vi "Main.vi"() -> ()   [LabVIEW 2023]
panel:
  in  "Start":bool
  in  "Vipassana Time (min)":dbl
  in  "Anapana Time (min)":dbl
  in  "Vipassana":bool
  in  "Anapana":bool
  # "Time(minutes)"
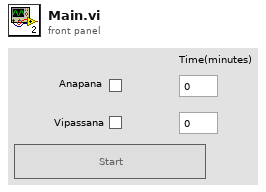
[diagram p1: front panel]
types:
  T1 = enum8{"Enabled", "Disabled", "Disabled and Grayed Out"}
  T2 = enum32{"Invalid", "Standard", "Closed", "Hidden", "Minimized", "Maximized"}
  T3 = enum32{"invalid app kind", "Development System", "Run Time System", "Student Edition", "Embedded LabVIEW", "Evaluation", "Custom"}
  T4 = cluster{"Core":cluster{"Current VI Reference":refnum<vi>, "Close Panel on Exit?":bool}, "Anapana Start Time":timestamp, "Vipassana Start Time":timestamp, "Anapana":bool, " Vipassana":bool, "Anapana Time (min)":dbl, "Vipassana Time (min)":dbl, "Real Sound?":bool}
  T5 = cluster{"Current VI Reference":refnum<vi>, "Close Panel on Exit?":bool}
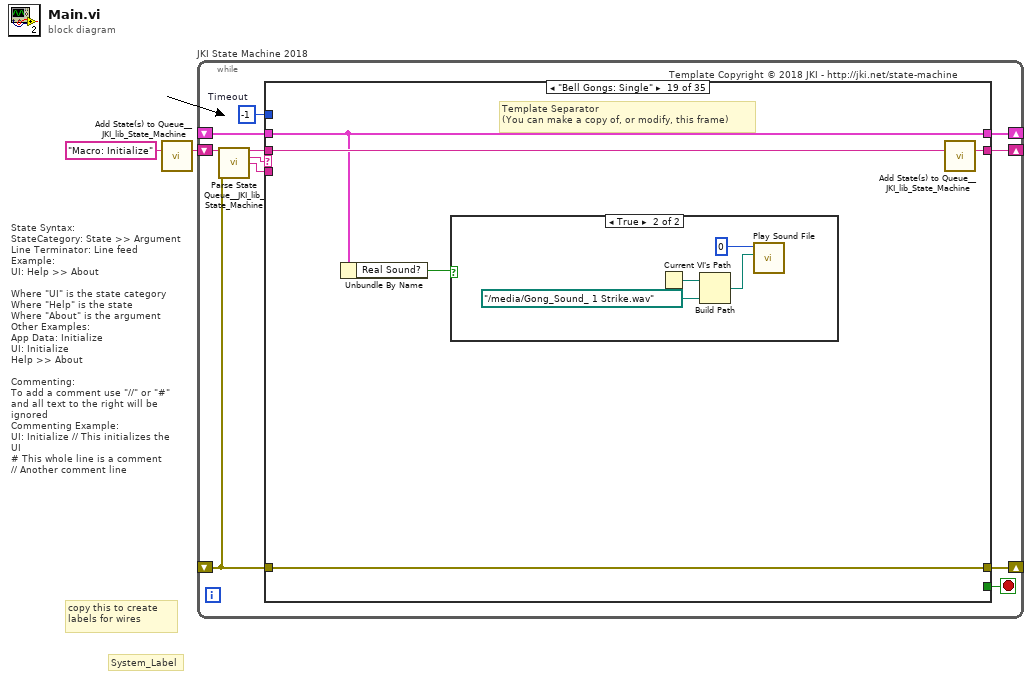
[diagram p0: block diagram]
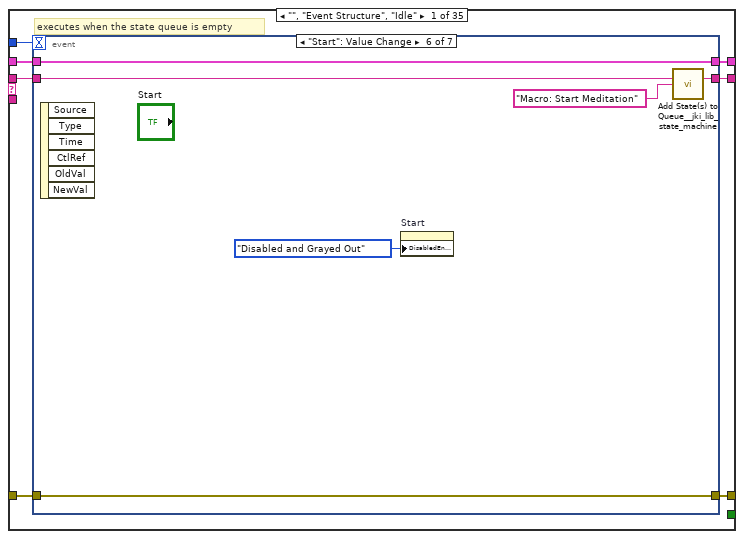
[diagram p2: hidden frame]
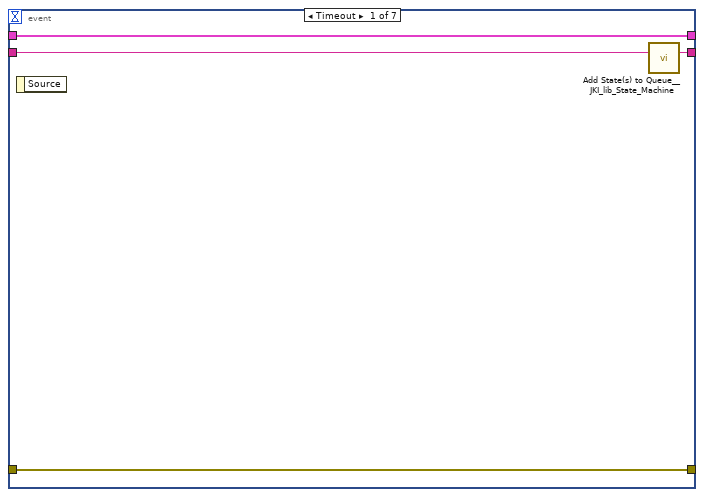
[diagram p3: hidden frame]
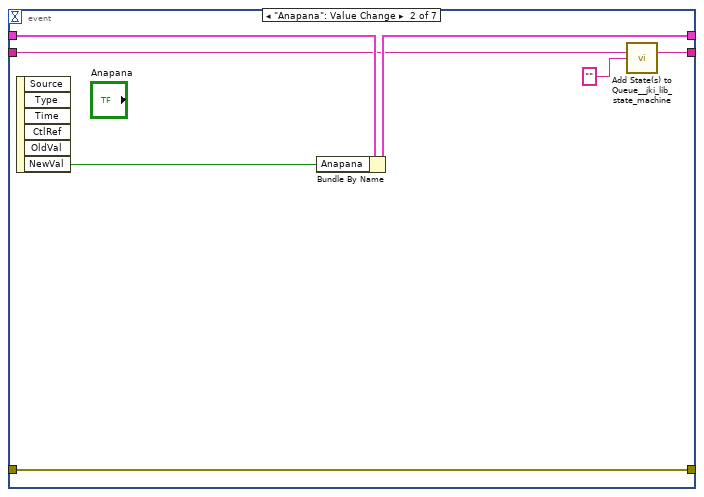
[diagram p4: hidden frame]
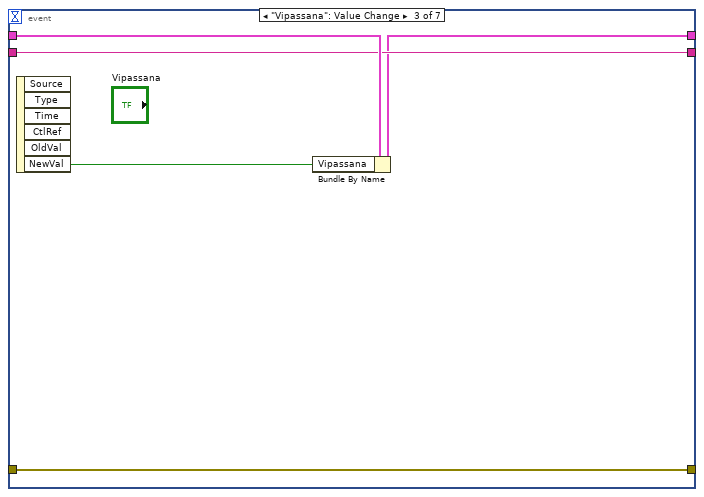
[diagram p5: hidden frame]
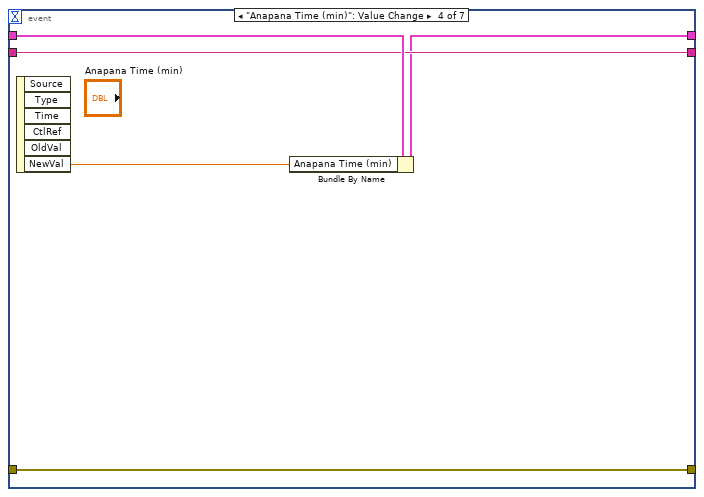
[diagram p6: hidden frame]
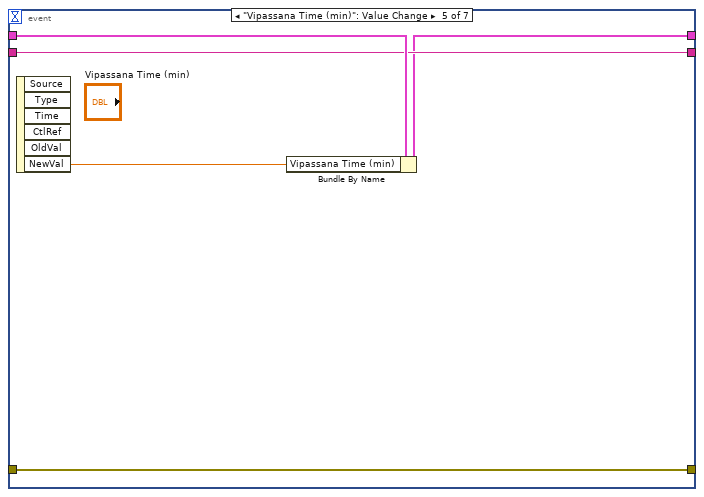
[diagram p7: hidden frame]
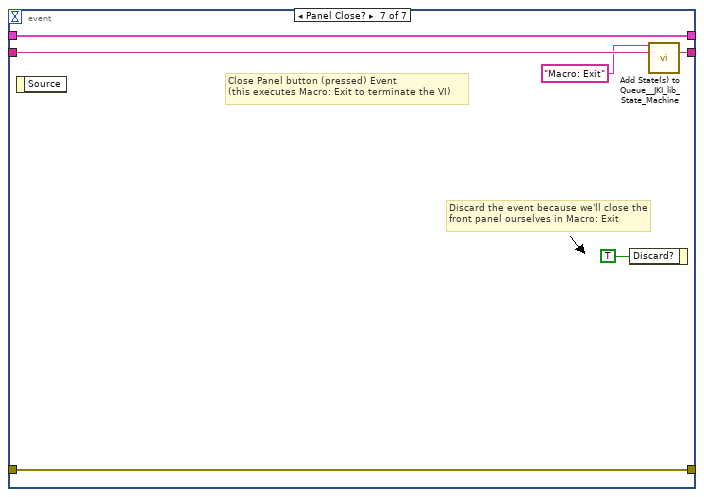
[diagram p8: hidden frame]
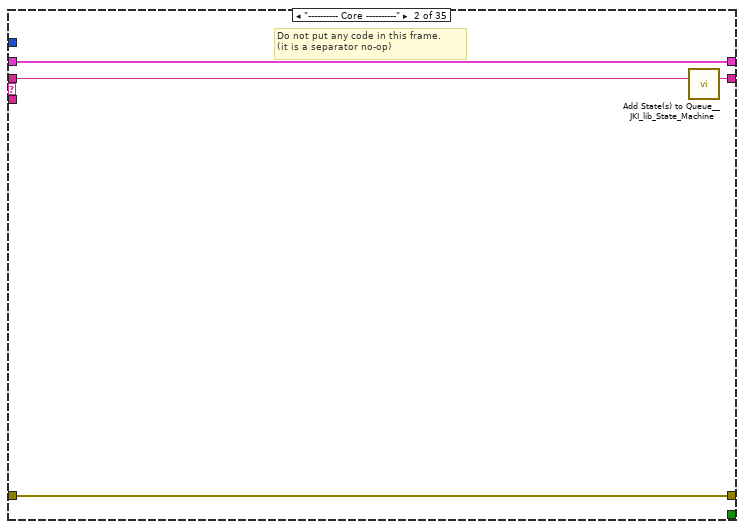
[diagram p9: hidden frame]
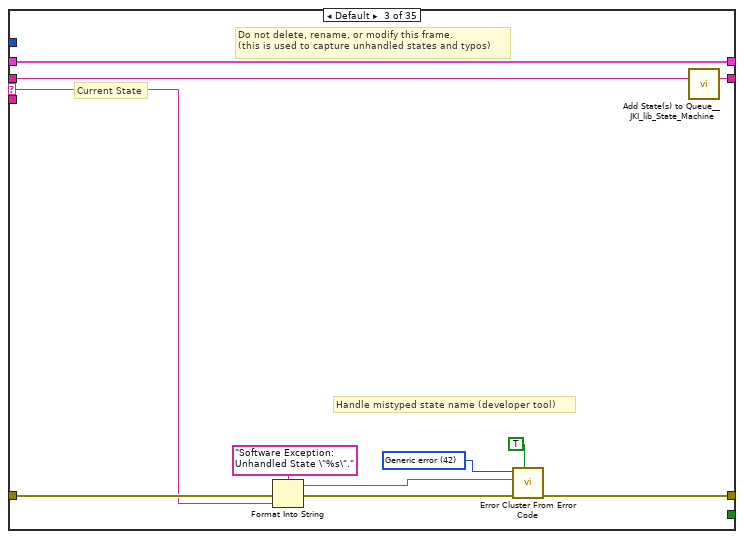
[diagram p10: hidden frame]
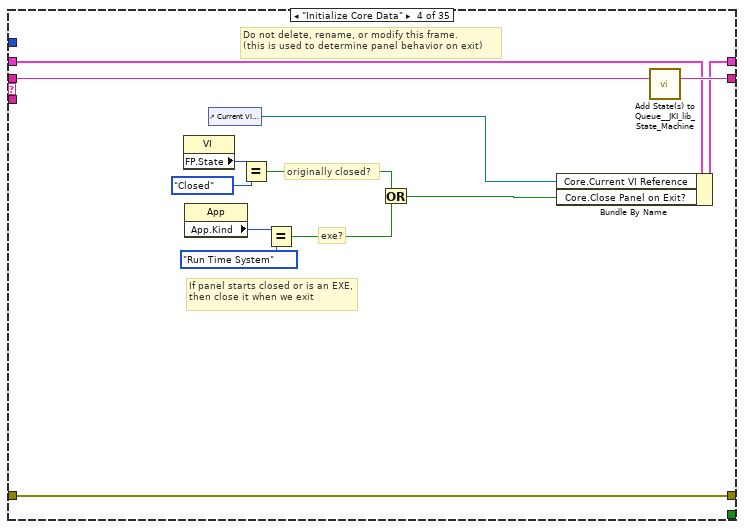
[diagram p11: hidden frame]
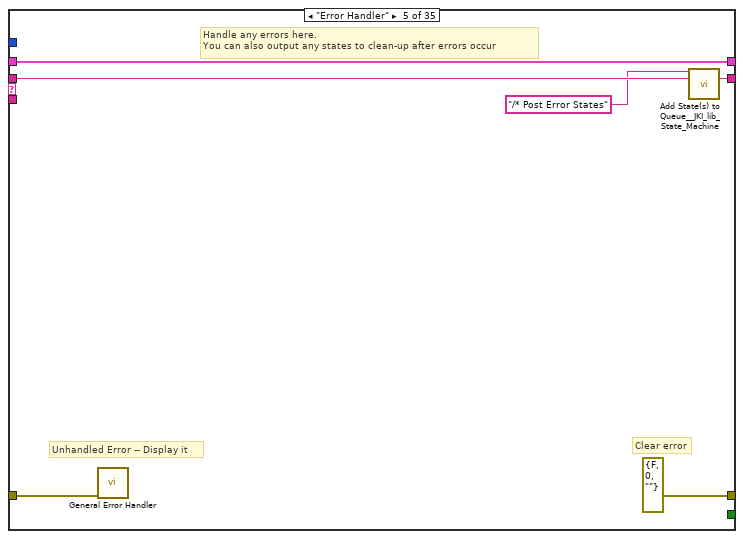
[diagram p12: hidden frame]
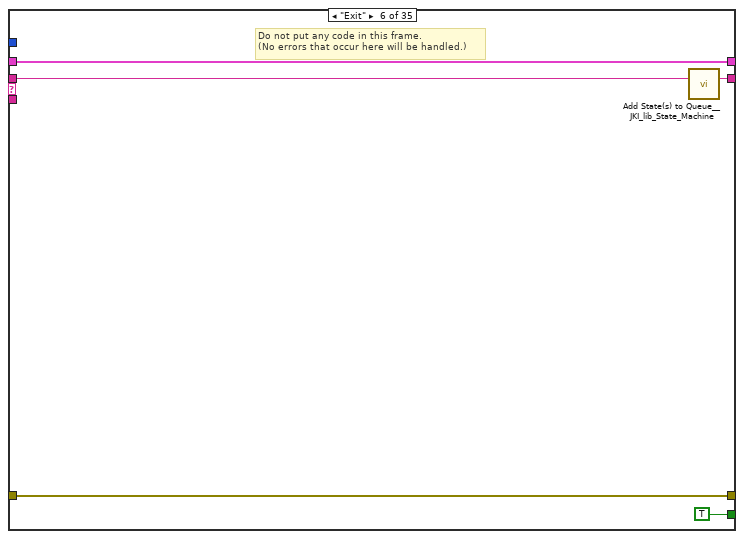
[diagram p13: hidden frame]
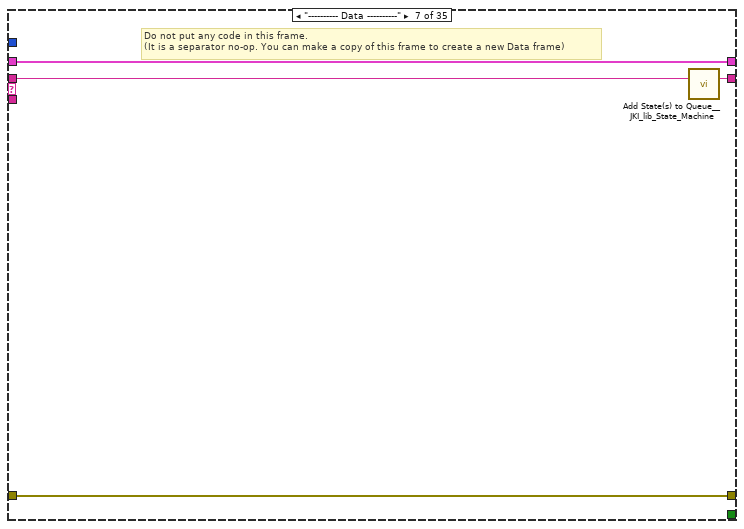
[diagram p14: hidden frame]
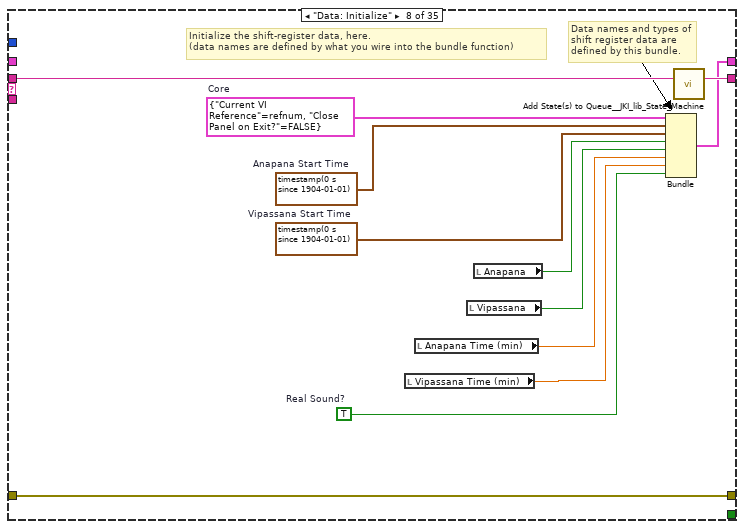
[diagram p15: hidden frame]
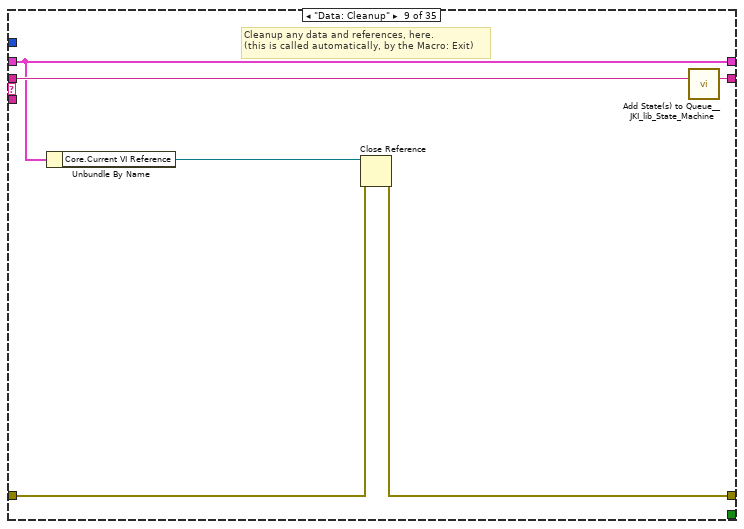
[diagram p16: hidden frame]
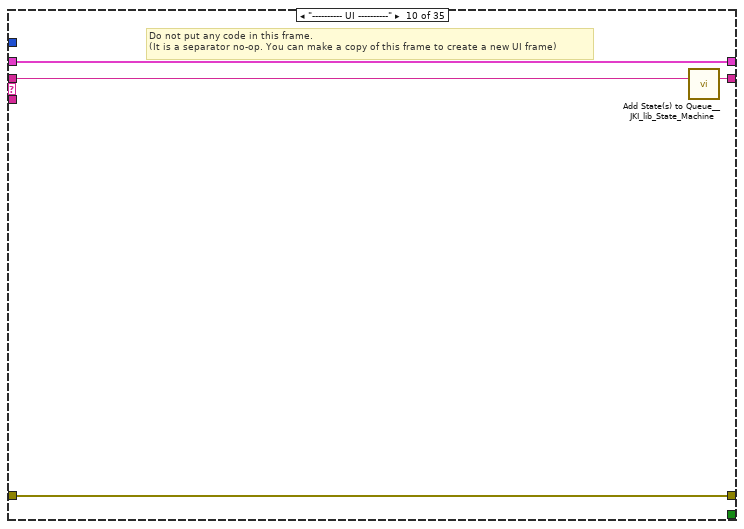
[diagram p17: hidden frame]
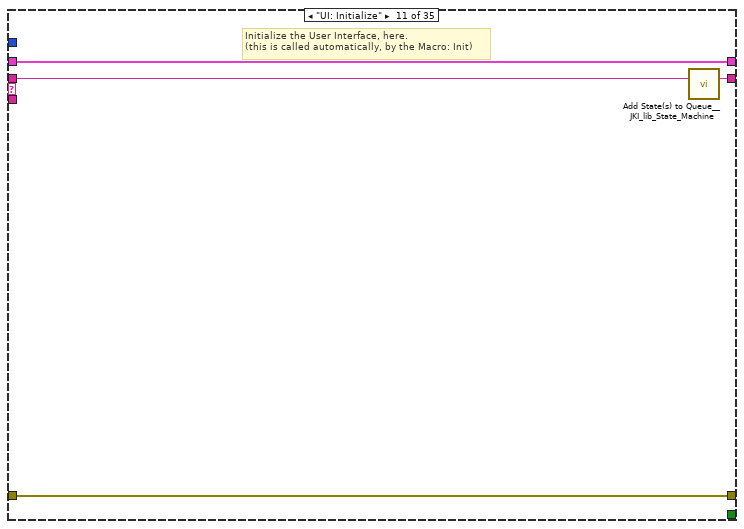
[diagram p18: hidden frame]
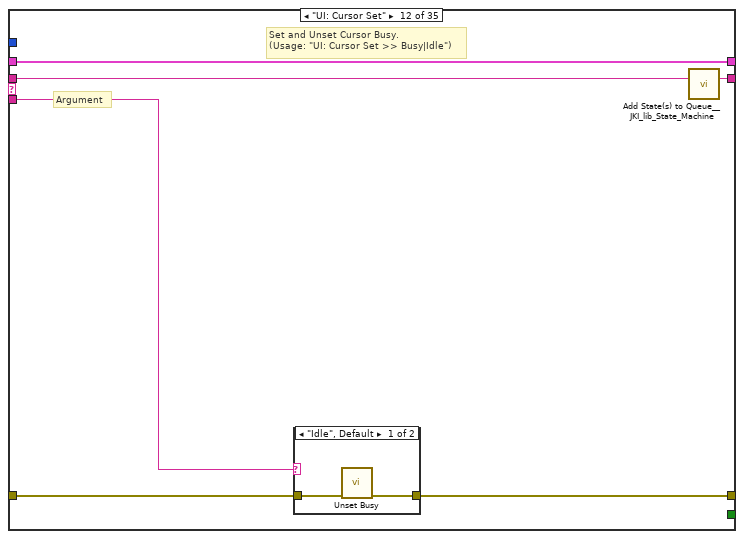
[diagram p19: hidden frame]
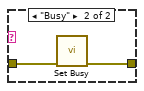
[diagram p20: hidden frame]
diagram:
  # "State Syntax:\nStateCategory: State >> Argument\nLine Terminator: Line feed\nExample:\nUI: Help >> About\n\nWhere \"UI\" is the state category\nWhere \"Help\" is the state\nWhere \"About\" is the argument\nOther Examples:\nApp Data: Initialize\nUI: Initialize\nHelp >> About\n\nCommenting:\nTo add a comment use \"//\" or \"#\" and all text to the right will be ignored\nCommenting Example:\nUI: Initialize // This initializes the UI\n# This whole line is a comment\n// Another comment line"
  # "copy this to create labels for wires"
  # "System_Label"
  n1 = call <vilib>:"Add State(s) to Queue__JKI_lib_State_Machine.vi"("State(s) in (\"\")"="Macro: Initialize") -> ("States Out"=w2:string)  [unwired: 14 in]
  n2 = while "JKI State Machine 2018" {
    shift-right: [w6] -> _
    shift-left: _ -> [w5]
    shift-right: [w9] -> _
    shift-left: _ -> [w3]
    shift-right: [w8] -> _
    shift-left: w2 -> [w10]
    stop <- w7 stop-if-true
    w4 = -1  # Timeout
    # "Template Copyright © 2018 JKI - http://jki.net/state-machine"
    n3 = call <vilib>:"Parse State Queue__JKI_lib_State_Machine.vi"("State Queue"=w10, "Error In (no error)"=w3) -> ("Remaining States"=w12:string, "Current State"=w13:string, "Arguments"=w11:string)  [unwired: 11 in]
    n4 = case shown="\"Bell Gongs: Single\"" w13 {
      selector: w13 -> [_ _ w63 _ _ _ _ _ _ _ _ _ _ _ _ _ _ _ _ _ _ _ _ _ _ _ _ _ _ _ _ _ _ _ _]
      tunnel: w12 -> [w20 w62 w67 w86 w92 w97 w101 w113 w119 w123 w127 w133 w144 w213 w219 w230 w240 w244 w249 w259 w268 w275 w291 w300 w306 w310 w321 w337 w342 w348 w352 w358 w381 w385 w390]
      tunnel: w11 -> [_ _ _ _ _ _ _ _ _ _ _ w128 w138 _ _ _ _ _ _ _ _ _ _ _ _ _ _ _ _ _ _ _ _ _ _]
      tunnel: w5 -> [w18 w59 w65 w79 w89 w95 w98 _ w114 w120 w125 w131 w140 w210 w216 w226 w237 w241 w246 w256 w265 w272 w281 w294 w303 w307 w314 w323 w339 w345 w349 w355 w378 w382 w387]
      tunnel: [w17 w60 w69 w83 errorcluster {"status"=FALSE, "code"=0, "source"=""} ("error out") w94 w99 w110 w115 w121 w124 w129 w141 w211 w217 w228 w238 w242 w247 w257 w266 w273 w289 w298 w304 w308 w319 w335 w340 w346 w350 w356 w379 w383 w388] -> w9
      tunnel: w3 -> [w16 w60 w68 w83 w88 w94 w99 w110 w116 w121 w124 w130 w142 w211 w217 w228 w238 w242 w247 w257 w266 w273 w289 w298 w304 w308 w319 w335 w340 w346 w350 w356 w379 w383 w388]
      tunnel: [w19 w61 w66 w85 w91 w96 w100 w112 w118 w122 w126 w132 w143 w212 w218 w229 w239 w243 w248 w258 w267 w274 w290 w299 w305 w309 w320 w336 w341 w347 w351 w357 w380 w384 w389] -> w8
      tunnel: [_ _ _ _ _ TRUE _ _ _ _ _ _ _ _ _ _ _ _ _ _ _ _ _ _ _ _ _ _ _ _ _ _ _ _ _] -> w7
      tunnel: [w15 w59 w65 w84 w89 w95 w98 w111 w114 w120 w125 w131 w140 w210 w216 w226 w237 w241 w246 w256 w265 w271 w281 w294 w303 w307 w317 w323 w339 w345 w349 w354 w378 w382 w387] -> w6
      tunnel: w4 -> [w14 _ _ _ _ _ _ _ _ _ _ _ _ _ _ _ _ _ _ _ _ _ _ _ _ _ _ _ _ _ _ _ _ _ _]
      frame "", "Event Structure", "Idle" {
        # "executes when the state queue is empty"
        n5 = event shown="[5] \"Start\": Value Change" {
          selector: _ -> [_ _ _ _ _ _ _]
          dyn-events: _ -> [_ _ _ _ _ _ _]
          timeout: w14 -> [_ _ _ _ _ _ _]
          tunnel: w20 -> [w24 w26 w35 w40 w45 w49 w58]
          tunnel: [w23 w27 w35 w40 w45 w50 w57] -> w19
          tunnel: w18 -> [w21 w31 w36 w41 w46 w52 w55]
          tunnel: [w22 w28 w32 w37 w42 w51 w56] -> w17
          tunnel: w16 -> [w22 w28 w32 w37 w42 w51 w56]
          tunnel: [w21 w30 w34 w39 w44 w52 w55] -> w15
          event Timeout {
            n6 = event-data() -> ()  [unwired: 1 in, 1 out]
            n7 = call <vilib>:"Add State(s) to Queue__JKI_lib_State_Machine.vi"("State(s) in (\"\")"=w24) -> ("States Out"=w23:string)  [unwired: 14 in]
          }
          event "Anapana": Value Change {
            n8 = event-data() -> ("NewVal"=w29:bool)  [unwired: 1 in, 5 out]
            n9 = Bundle By Name(cluster=w31, "Anapana"=w29) -> (w30:T4)
            n10 = call <vilib>:"Add State(s) to Queue__jki_lib_state_machine.vi"("State(s) in (\"\")"=w26, "State(s) at Back (\"\")"="" ("State(s) at Back (\"\")")) -> ("States Out"=w27:string)  [unwired: 13 in]
          }
          event "Vipassana": Value Change {
            n11 = event-data() -> ("NewVal"=w33:bool)  [unwired: 1 in, 5 out]
            n12 = Bundle By Name(cluster=w36, "Vipassana"=w33) -> (w34:T4)
          }
          event "Anapana Time (min)": Value Change {
            n13 = event-data() -> ("NewVal"=w38:dbl)  [unwired: 1 in, 5 out]
            n14 = Bundle By Name(cluster=w41, "Anapana Time (min)"=w38) -> (w39:T4)
          }
          event "Vipassana Time (min)": Value Change {
            n15 = event-data() -> ("NewVal"=w43:dbl)  [unwired: 1 in, 5 out]
            n16 = Bundle By Name(cluster=w46, "Vipassana Time (min)"=w43) -> (w44:T4)
          }
          event "Start": Value Change {
            n17 = event-data() -> ()  [unwired: 1 in, 6 out]
            n18 = property on="Start" class="Bool"("DisabledEnum"=T1."Disabled and Grayed Out" ("Disabled")) -> ()  [unwired: 2 in, 2 out]
            n19 = call <vilib>:"Add State(s) to Queue__jki_lib_state_machine.vi"("State(s) in (\"\")"=w49, "State(s) at Back (\"\")"="Macro: Start Meditation" ("State(s) at Back (\"\")")) -> ("States Out"=w50:string)  [unwired: 13 in]
          }
          event Panel Close? {
            # "Discard the event because we'll close the front panel ourselves in Macro: Exit"
            # "Close Panel button (pressed) Event\n(this executes Macro: Exit to terminate the VI)"
            n20 = event-data() -> ()  [unwired: 1 in, 1 out]
            n21 = event-data("Discard?"=TRUE) -> ()  [unwired: 1 in, 1 out]
            n22 = call <vilib>:"Add State(s) to Queue__JKI_lib_State_Machine.vi"("State(s) in Front (\"\")"="Macro: Exit", "State(s) in (\"\")"=w58) -> ("States Out"=w57:string)  [unwired: 13 in]
          }
        }
      }
      frame "---------- Core ----------" {
        # "Do not put any code in this frame.\n(it is a separator no-op)"
        n23 = call <vilib>:"Add State(s) to Queue__JKI_lib_State_Machine.vi"("State(s) in (\"\")"=w62) -> ("States Out"=w61:string)  [unwired: 14 in]
      }
      frame Default {
        w72 = 42 items=["No error", "Argument error", "Memory is full", "Out of zone", "End of file", "File already open", "Generic file I/O error", "File not found", "File permission error", "Disk is full", "Duplicate path", "Too many files open", "System feature not enabled", "Resource file not found", "Cannot add resource", "Resource not found", "Image not found", "Image memory error", "Pen does not exist", "Config type invalid", "Config token not found", "Config parse error", "Config memory error", "Bad external code format", "Bad external code offset", "External code not present", "Null window", "Destroy window error", "Null menu", "Print aborted", "Bad print record", "Print driver error", "Windows error during printing", "Memory error during printing", "Print dialog error", "Generic print error", "Invalid device refnum", "Device not found", "Device parameter error", "Device unit error", "Cannot open device", "Device call aborted", "Generic error", "Cancelled by user", "Object ID too low", "Object ID too high", "Object not in heap", "Unknown heap", "Unknown object (invalid DefProc)", "Unknown object (DefProc not in table)", "Message out of range", "Invalid (null) method", "Unknown message", "Manager call not supported", "Bad address", "Network operation in progress", "Network operation timed out", "Connection is busy", "Network attribute not supported", "Network error", "Address in use", "System out of memory", "Connection aborted", "Connection refused", "Not connected", "Already connected", "Connection closed", "Initialization error (interapplication manager)", "Bad occurrence", "Wait on unbound occurrence handler", "Occurrence queue overflow", "Datalog type conflict", "Unused", "Unrecognized type (interapplication manager)", "Memory corrupt", "Failed to make temporary DLL", "Old CIN version", "Drag socket not found", "Failed to load drop-object", "Failed to register OLE object", "Failed to release OLE object", "Format specifier type mismatch", "Unknown format specifier", "Too few format specifiers", "Too many format specifiers", "Scan failed", "Newer CIN version", "Error converting to variant", "Runtime menu error", "Password tampered", "Variant attribute not found", "Incompatible variant data type", "Event data is not available", "Event Store is not present", "Occurrence is not found", "Event Queue is not created", "Event info is not available", "Refnum passed is NULL", "Error retrieving Class GUID", "Error retrieving CoClass GUID", "Error retrieving TypeLib GUID.", "Bad built application magic bytes.", "Specific driver is different from the specific driver associated with the Logical Name.", "There is no session opened to the class driver.", "Max Error", "MAX - Error with config objects", "MAX - Error loading configuration", "MAX - Group not supported"]
        # "Current State"
        # "Do not delete, rename, or modify this frame.\n(this is used to capture unhandled states and typos)"
        # "Handle mistyped state name (developer tool)"
        n24 = Format Into String(format string="Software Exception: Unhandled State \"%s\"." ("message"), error in=w68, w63) -> (resulting string=w71:string, error out=w70:errorcluster)  [unwired: 1 in]
        n25 = call <vilib>:"Error Cluster From Error Code.vi"("show call chain? (False)"=TRUE, "error in (no error)"=w70, "error message (\"\")"=w71, "error code (0)"=w72) -> ("error out"=w69:errorcluster)  [unwired: 5 in]
        n26 = call <vilib>:"Add State(s) to Queue__JKI_lib_State_Machine.vi"("State(s) in (\"\")"=w67) -> ("States Out"=w66:string)  [unwired: 14 in]
      }
      frame "Initialize Core Data" {
        # "Do not delete, rename, or modify this frame.\n(this is used to determine panel behavior on exit)"
        # "originally closed?"
        # "exe?"
        # "If panel starts closed or is an EXE, then close it when we exit"
        n27 = property class="VI"() -> ("FP.State"=w76:T2)  [unwired: 2 in, 2 out]
        n28 = property class="App"() -> ("App.Kind"=w82:T3)  [unwired: 2 in, 2 out]
        n29 = control-ref of="Current VI Reference"() -> (w77:refnum<vi>)
        n30 = Equal?(x=w76, y=T2."Closed" ("Front Panel Window:State")) -> (x = y?=w74:bool)
        n31 = Equal?(x=w82, y=T3."Run Time System" ("Application:Kind")) -> (x = y?=w80:bool)
        n32 = Or(x=w74, y=w80) -> (x .or. y?=w78:bool)
        n33 = Bundle By Name(cluster=w79, "Core.Current VI Reference"=w77, "Core.Close Panel on Exit?"=w78) -> (w84:T4)
        n34 = call <vilib>:"Add State(s) to Queue__JKI_lib_State_Machine.vi"("State(s) in (\"\")"=w86) -> ("States Out"=w85:string)  [unwired: 14 in]
      }
      frame "Error Handler" {
        # "Unhandled Error -- Display it"
        # "Handle any errors here.\nYou can also output any states to clean-up after errors occur"
        # "Clear error"
        n35 = call <vilib>:"General Error Handler.vi"("error in (no error)"=w88) -> ()  [unwired: 10 in, 5 out]
        n36 = call <vilib>:"Add State(s) to Queue__JKI_lib_State_Machine.vi"("State(s) in Front (\"\")"="/* Post Error States", "State(s) in (\"\")"=w92) -> ("States Out"=w91:string)  [unwired: 13 in]
      }
      frame "Exit" {
        # "Do not put any code in this frame.\n(No errors that occur here will be handled.)"
        n37 = call <vilib>:"Add State(s) to Queue__JKI_lib_State_Machine.vi"("State(s) in (\"\")"=w97) -> ("States Out"=w96:string)  [unwired: 14 in]
      }
      frame "---------- Data ----------" {
        # "Do not put any code in this frame.\n(It is a separator no-op. You can make a copy of this frame to create a new Data frame)"
        n38 = call <vilib>:"Add State(s) to Queue__JKI_lib_State_Machine.vi"("State(s) in (\"\")"=w101) -> ("States Out"=w100:string)  [unwired: 14 in]
      }
      frame "Data: Initialize" {
        w106 = TRUE  # Real Sound?
        w107 = timestamp(0 s since 1904-01-01)  # Vipassana Start Time
        w108 = timestamp(0 s since 1904-01-01)  # Anapana Start Time
        w109 = T5 {"Current VI Reference"=refnum, "Close Panel on Exit?"=FALSE}  # Core
        # "Data names and types of shift register data are defined by this bundle."
        # "Initialize the shift-register data, here.\n(data names are defined by what you wire into the bundle function)"
        n39 = local read "Vipassana Time (min)"() -> (w102:dbl)
        n40 = local read "Anapana Time (min)"() -> (w103:dbl)
        n41 = local read "Vipassana"() -> (w104:bool)
        n42 = local read "Anapana"() -> (w105:bool)
        n43 = Bundle("Core"=w109, "Anapana Start Time"=w108, "Vipassana Start Time"=w107, "Anapana"=w105, "Vipassana"=w104, "Anapana Time (min)"=w103, "Vipassana Time (min)"=w102, "Real Sound?"=w106) -> (w111:T4)  [unwired: 1 in]
        n44 = call <vilib>:"Add State(s) to Queue__JKI_lib_State_Machine.vi"("State(s) in (\"\")"=w113) -> ("States Out"=w112:string)  [unwired: 14 in]
      }
      frame "Data: Cleanup" {
        # "Cleanup any data and references, here.\n(this is called automatically, by the Macro: Exit)"
        n45 = Unbundle By Name(w114) -> ("Core.Current VI Reference"=w117:refnum<vi>)
        n46 = Close Reference(reference=w117, error in (no error)=w116) -> (error out=w115:errorcluster)
        n47 = call <vilib>:"Add State(s) to Queue__JKI_lib_State_Machine.vi"("State(s) in (\"\")"=w119) -> ("States Out"=w118:string)  [unwired: 14 in]
      }
      frame "---------- UI ----------" {
        # "Do not put any code in this frame.\n(It is a separator no-op. You can make a copy of this frame to create a new UI frame)"
        n48 = call <vilib>:"Add State(s) to Queue__JKI_lib_State_Machine.vi"("State(s) in (\"\")"=w123) -> ("States Out"=w122:string)  [unwired: 14 in]
      }
      frame "UI: Initialize" {
        # "Initialize the User Interface, here.\n(this is called automatically, by the Macro: Init)"
        n49 = call <vilib>:"Add State(s) to Queue__JKI_lib_State_Machine.vi"("State(s) in (\"\")"=w127) -> ("States Out"=w126:string)  [unwired: 14 in]
      }
      frame "UI: Cursor Set" {
        # "Argument"
        # "Set and Unset Cursor Busy.\n(Usage: \"UI: Cursor Set >> Busy|Idle\")"
        n50 = case shown="\"Idle\", Default" w128 {
          tunnel: w130 -> [w135 w137]
          tunnel: [w134 w136] -> w129
          frame "Idle", Default {
            n51 = call <vilib>:"Unset Busy.vi"("error in (no error)"=w135) -> ("error out"=w134:errorcluster)  [unwired: 10 in]
          }
          frame "Busy" {
            n52 = call <vilib>:"Set Busy.vi"("error in (no error)"=w137) -> ("error out"=w136:errorcluster)  [unwired: 9 in, 1 out]
          }
        }
        n53 = call <vilib>:"Add State(s) to Queue__JKI_lib_State_Machine.vi"("State(s) in (\"\")"=w133) -> ("States Out"=w132:string)  [unwired: 14 in]
      }
      frame "UI: Front Panel State" {
        # "Argument"
        # "Set Front Panel Open or Closed\n(Usage: \"UI: Front Panel State >> Open|Close\")"
        n54 = Unbundle By Name(w140) -> ("Core.Current VI Reference"=w139:refnum<vi>)
        n55 = case shown="\"Minimize\", \"Minimized\"" w138 {
          tunnel: w142 -> [w150 w165 w176 w189 w202]
          tunnel: [w152 w166 w178 w191 w204] -> w141
          tunnel: w139 -> [w151 w163 w177 w190 w203]
          frame "Open", "Standard", Default {
            w145 = T2."Standard" ("State")
            n56 = property class="VI"(reference=w151, error in=w150) -> (reference out=w148:refnum<vi>, error out=w149:errorcluster, "FP.State"=w147:T2)
            n57 = Not Equal?(x=w147, y=w145) -> (x != y?=w146:bool)
            n58 = case shown="True" w146 {
              tunnel: [w156 w158] -> w152
              tunnel: w149 -> [w155 w158]
              tunnel: w148 -> [w154 _]
              tunnel: w145 -> [w153 _]
              frame True {
                n59 = invoke class="VI" method="FP.Open"(reference=w154, error in=w155, "Activate"=TRUE, "State"=w153) -> (error out=w156:errorcluster)  [unwired: 1 in, 4 out]
              }
              frame False {
              }
            }
          }
          frame "Close", "Closed" {
            n60 = property class="VI"(reference=w163, error in=w165) -> (reference out=w162:refnum<vi>, error out=w164:errorcluster, "FP.State"=w160:T2)
            n61 = Not Equal?(x=w160, y=T2."Closed" ("Front Panel Window:State")) -> (x != y?=w159:bool)
            n62 = case shown="True" w159 {
              tunnel: [w167 w170] -> w166
              tunnel: w164 -> [w167 w169]
              tunnel: w162 -> [_ w168]
              frame False {
              }
              frame True {
                n63 = invoke class="VI" method="FP.Close"(reference=w168, error in=w169) -> (error out=w170:errorcluster)  [unwired: 1 in, 2 out]
              }
            }
          }
          frame "Hidden", "Hide" {
            w171 = T2."Hidden" ("State")
            n64 = property class="VI"(reference=w177, error in=w176) -> (reference out=w174:refnum<vi>, error out=w175:errorcluster, "FP.State"=w173:T2)
            n65 = Not Equal?(x=w173, y=w171) -> (x != y?=w172:bool)
            n66 = case shown="True" w172 {
              tunnel: [w182 w183] -> w178
              tunnel: w175 -> [w181 w183]
              tunnel: w174 -> [w180 _]
              tunnel: w171 -> [w179 _]
              frame True {
                n67 = invoke class="VI" method="FP.Open"(reference=w180, error in=w181, "State"=w179) -> (error out=w182:errorcluster)  [unwired: 2 in, 4 out]
              }
              frame False {
              }
            }
          }
          frame "Minimize", "Minimized" {
            w184 = T2."Minimized" ("State")
            n68 = property class="VI"(reference=w190, error in=w189) -> (reference out=w187:refnum<vi>, error out=w188:errorcluster, "FP.State"=w186:T2)
            n69 = Not Equal?(x=w186, y=w184) -> (x != y?=w185:bool)
            n70 = case shown="True" w185 {
              tunnel: [w195 w196] -> w191
              tunnel: w188 -> [w194 w196]
              tunnel: w187 -> [w193 _]
              tunnel: w184 -> [w192 _]
              frame True {
                n71 = invoke class="VI" method="FP.Open"(reference=w193, error in=w194, "State"=w192) -> (error out=w195:errorcluster)  [unwired: 2 in, 4 out]
              }
              frame False {
              }
            }
          }
          frame "Maximize", "Maximized" {
            w197 = T2."Maximized" ("State")
            n72 = property class="VI"(reference=w203, error in=w202) -> (reference out=w200:refnum<vi>, error out=w201:errorcluster, "FP.State"=w199:T2)
            n73 = Not Equal?(x=w199, y=w197) -> (x != y?=w198:bool)
            n74 = case shown="True" w198 {
              tunnel: [w208 w209] -> w204
              tunnel: w201 -> [w207 w209]
              tunnel: w200 -> [w206 _]
              tunnel: w197 -> [w205 _]
              frame True {
                n75 = invoke class="VI" method="FP.Open"(reference=w206, error in=w207, "State"=w205) -> (error out=w208:errorcluster)  [unwired: 2 in, 4 out]
              }
              frame False {
              }
            }
          }
        }
        n76 = call <vilib>:"Add State(s) to Queue__JKI_lib_State_Machine.vi"("State(s) in (\"\")"=w144) -> ("States Out"=w143:string)  [unwired: 14 in]
      }
      frame "---------- Macro ----------" {
        # "Do not put any code in this frame.\n(It is a separator no-op. You can make a copy of this frame to create a new Macro frame)"
        n77 = call <vilib>:"Add State(s) to Queue__JKI_lib_State_Machine.vi"("State(s) in (\"\")"=w213) -> ("States Out"=w212:string)  [unwired: 14 in]
      }
      frame "Macro: Initialize" {
        w215 = "Data: Initialize\nInitialize Core Data\nUI: Initialize\nUI: Front Panel State >> Open"  # Data: Initialize Initialize Core Data UI: Initialize UI: Front Panel State >> Open
        # "Initialization Macro\n(This is called once, when the VI starts)"
        n78 = property on="Start" class="Bool"("DisabledEnum"=T1."Enabled" ("Disabled")) -> ()  [unwired: 2 in, 2 out]
        n79 = call <vilib>:"Add State(s) to Queue__JKI_lib_State_Machine.vi"("State(s) in Front (\"\")"=w215, "State(s) in (\"\")"=w219) -> ("States Out"=w218:string)  [unwired: 13 in]
      }
      frame "Macro: Start Meditation" {
        # "Initialization Macro\n(This is called once, when the VI starts)"
        n80 = Unbundle By Name(w226) -> ("Anapana"=w224:bool, "Vipassana"=w221:bool)
        n81 = Select(t="Vipassana: Start\nVipassana: Check", s=w221, f="") -> (s? t:f=w220:string)
        n82 = Select(t="Anapana: Start\nAnapana: Check", s=w224, f=w220) -> (s? t:f=w225:string)
        n83 = call <vilib>:"Add State(s) to Queue__JKI_lib_State_Machine.vi"("State(s) in Front (\"\")"=w225, "State(s) in (\"\")"=w230) -> ("States Out"=w229:string)  [unwired: 13 in]
      }
      frame "Macro: Exit" {
        # "Exit Macro\n(This is called once, when the VI exits)"
        n84 = Unbundle By Name(w237) -> ("Core.Close Panel on Exit?"=w236:bool)
        n85 = Select(t="UI: Front Panel State >> Close", s=w236, f="") -> (s? t:f=w233:string)
        n86 = call <vilib>:"Add State(s) to Queue__JKI_lib_State_Machine.vi"("State(s) in (\"\")"=w233, "State(s) at Back (\"\")"="Data: Cleanup\nExit") -> ("States Out"=w231:string)  [unwired: 13 in]
        n87 = call <vilib>:"Add State(s) to Queue__JKI_lib_State_Machine.vi"("State(s) in Front (\"\")"=w231, "State(s) in (\"\")"=w240) -> ("States Out"=w239:string)  [unwired: 13 in]
      }
      frame "---------- Bell Gongs ----------" {
        # "Template Separator\n(You can make a copy of, or modify, this frame)"
        n88 = call <vilib>:"Add State(s) to Queue__JKI_lib_State_Machine.vi"("State(s) in (\"\")"=w244) -> ("States Out"=w243:string)  [unwired: 14 in]
      }
      frame "Bell Gongs: Single" {
        # "Template Separator\n(You can make a copy of, or modify, this frame)"
        n89 = Unbundle By Name(w246) -> ("Real Sound?"=w245:bool)
        n90 = case shown="True" w245 {
          frame False {
            n91 = One Button Dialog(message="Single Dong") -> ()  [unwired: 1 in, 1 out]
          }
          frame True {
            n92 = Current VI's Path() -> (path=w251:path)
            n93 = Build Path(base path=w251, name or relative path=path "../media/Gong_Sound_ 1 Strike.wav" ("Sound File Path")) -> (appended path=w252:path)
            n94 = call <vilib>:"Play Sound File.vi"("path"=w252, "device ID"=u32 0 ("Device ID")) -> ()  [unwired: 8 in, 2 out]
          }
        }
        n95 = call <vilib>:"Add State(s) to Queue__JKI_lib_State_Machine.vi"("State(s) in (\"\")"=w249) -> ("States Out"=w248:string)  [unwired: 14 in]
      }
      frame "Bell Gongs: Tripple" {
        # "Template Separator\n(You can make a copy of, or modify, this frame)"
        n96 = Unbundle By Name(w256) -> ("Real Sound?"=w255:bool)
        n97 = case shown="False" w255 {
          frame False {
            n98 = One Button Dialog(message="Tripple Gong") -> ()  [unwired: 1 in, 1 out]
          }
          frame True {
            n99 = Current VI's Path() -> (path=w261:path)
            n100 = Build Path(base path=w261, name or relative path=path "../media/Gong_Sound_ 3 Strikes.wav" ("Sound File Path")) -> (appended path=w262:path)
            n101 = call <vilib>:"Play Sound File.vi"("path"=w262, "device ID"=u32 0 ("Device ID")) -> ()  [unwired: 8 in, 2 out]
          }
        }
        n102 = call <vilib>:"Add State(s) to Queue__JKI_lib_State_Machine.vi"("State(s) in (\"\")"=w259) -> ("States Out"=w258:string)  [unwired: 14 in]
      }
      frame "---------- Anapana ----------" {
        # "Template Separator\n(You can make a copy of, or modify, this frame)"
        n103 = call <vilib>:"Add State(s) to Queue__JKI_lib_State_Machine.vi"("State(s) in (\"\")"=w268) -> ("States Out"=w267:string)  [unwired: 14 in]
      }
      frame "Anapana: Start" {
        # "Template Separator\n(You can make a copy of, or modify, this frame)"
        n104 = Get Date/Time In Seconds() -> (seconds since 1Jan1904=w270:timestamp)
        n105 = Bundle By Name(cluster=w272, "Anapana Start Time"=w270) -> (w271:T4)
        n106 = call <vilib>:"Add State(s) to Queue__JKI_lib_State_Machine.vi"("State(s) in (\"\")"=w275, "State(s) at Back (\"\")"="Bell Gongs: Tripple" ("State(s) at Back (\"\")")) -> ("States Out"=w274:string)  [unwired: 13 in]
      }
      frame "Anapana: Check" {
        # "Template Separator\n(You can make a copy of, or modify, this frame)"
        n107 = Unbundle By Name(w281) -> ("Anapana Start Time"=w287:timestamp, "Anapana"=w283:bool, "Anapana Time (min)"=w286:dbl)
        n108 = Get Date/Time In Seconds() -> (seconds since 1Jan1904=w288:timestamp)
        n109 = Subtract(x=w288, y=w287) -> (x-y=w282:dbl)
        n110 = Multiply(x=w286, y=60.0) -> (x*y=w285:dbl)
        n111 = Greater?(x=w282, y=w285) -> (0:w284:bool)
        n112 = And(x=w284, y=w283) -> (x .and. y?=w279:bool)
        n113 = Select(t="Anapana: Finish", s=w279, f="Anapana: Keep Meditate") -> (s? t:f=w277:string)
        n114 = call <vilib>:"Add State(s) to Queue__JKI_lib_State_Machine.vi"("State(s) in (\"\")"=w291, "State(s) at Back (\"\")"=w277) -> ("States Out"=w290:string)  [unwired: 13 in]
      }
      frame "Anapana: Finish" {
        # "Finish meditation if no vipassana\nwith three gong"
        # "Template Separator\n(You can make a copy of, or modify, this frame)"
        n115 = Unbundle By Name(w294) -> ("Vipassana"=w295:bool)
        n116 = Not(x=w295) -> (.not. x?=w293:bool)
        n117 = Select(t="Bell Gongs: Tripple", s=w293, f="Bell Gongs: Single") -> (s? t:f=w296:string)
        n118 = call <vilib>:"Add State(s) to Queue__JKI_lib_State_Machine.vi"("State(s) in (\"\")"=w300, "State(s) at Back (\"\")"=w296) -> ("States Out"=w299:string)  [unwired: 13 in]
      }
      frame "Anapana: Keep Meditate" {
        # "Your code here.\n(You can make a copy of, or modify, this frame)"
        n119 = Wait (ms)(milliseconds to wait=u32 100) -> ()  [unwired: 1 out]
        n120 = call <vilib>:"Add State(s) to Queue__JKI_lib_State_Machine.vi"("State(s) in (\"\")"=w306, "State(s) at Back (\"\")"="Anapana: Check" ("State(s) at Back (\"\")")) -> ("States Out"=w305:string)  [unwired: 13 in]
      }
      frame "---------- Vipassana ----------" {
        # "Template Separator\n(You can make a copy of, or modify, this frame)"
        n121 = call <vilib>:"Add State(s) to Queue__JKI_lib_State_Machine.vi"("State(s) in (\"\")"=w310) -> ("States Out"=w309:string)  [unwired: 14 in]
      }
      frame "Vipassana: Start" {
        # "Start meditation with three three\ngongs if no anapana in begging"
        # "Template Separator\n(You can make a copy of, or modify, this frame)"
        n122 = Unbundle By Name(w314) -> ("Anapana"=w315:bool)
        n123 = Get Date/Time In Seconds() -> (seconds since 1Jan1904=w318:timestamp)
        n124 = Bundle By Name(cluster=w314, "Vipassana Start Time"=w318) -> (w317:T4)
        n125 = Not(x=w315) -> (.not. x?=w313:bool)
        n126 = Select(t="Bell Gongs: Tripple", s=w313, f="") -> (s? t:f=w311:string)
        n127 = call <vilib>:"Add State(s) to Queue__JKI_lib_State_Machine.vi"("State(s) in (\"\")"=w321, "State(s) at Back (\"\")"=w311) -> ("States Out"=w320:string)  [unwired: 13 in]
      }
      frame "Vipassana: Check" {
        # "Template Separator\n(You can make a copy of, or modify, this frame)"
        n128 = Unbundle By Name(w323) -> ("Vipassana Start Time"=w333:timestamp, "Vipassana"=w329:bool, "Vipassana Time (min)"=w332:dbl)
        n129 = Get Date/Time In Seconds() -> (seconds since 1Jan1904=w334:timestamp)
        n130 = Subtract(x=w334, y=w333) -> (x-y=w328:dbl)
        n131 = Multiply(x=w332, y=60.0) -> (x*y=w331:dbl)
        n132 = Greater?(x=w328, y=w331) -> (0:w330:bool)
        n133 = And(x=w330, y=w329) -> (x .and. y?=w326:bool)
        n134 = Select(t="Vipassana: Finish", s=w326, f="Vipassana: Keep Meditate") -> (s? t:f=w322:string)
        n135 = call <vilib>:"Add State(s) to Queue__JKI_lib_State_Machine.vi"("State(s) in (\"\")"=w337, "State(s) at Back (\"\")"=w322) -> ("States Out"=w336:string)  [unwired: 13 in]
      }
      frame "Vipassana: Finish" {
        # "Template Separator\n(You can make a copy of, or modify, this frame)"
        n136 = call <vilib>:"Add State(s) to Queue__JKI_lib_State_Machine.vi"("State(s) in (\"\")"=w342, "State(s) at Back (\"\")"="Bell Gongs: Tripple") -> ("States Out"=w341:string)  [unwired: 13 in]
      }
      frame "Vipassana: Keep Meditate" {
        # "Your code here.\n(You can make a copy of, or modify, this frame)"
        n137 = Wait (ms)(milliseconds to wait=u32 100) -> ()  [unwired: 1 out]
        n138 = call <vilib>:"Add State(s) to Queue__JKI_lib_State_Machine.vi"("State(s) in (\"\")"=w348, "State(s) at Back (\"\")"="Vipassana: Check" ("State(s) at Back (\"\")")) -> ("States Out"=w347:string)  [unwired: 13 in]
      }
      frame "---------- Timers ----------" {
        # "Template Separator\n(You can make a copy of, or modify, this frame)"
        n139 = call <vilib>:"Add State(s) to Queue__JKI_lib_State_Machine.vi"("State(s) in (\"\")"=w352) -> ("States Out"=w351:string)  [unwired: 14 in]
      }
      frame "Timer: Start" {
        # "Your code here.\n(You can make a copy of, or modify, this frame)"
        n140 = Get Date/Time In Seconds() -> (seconds since 1Jan1904=w353:timestamp)
        n141 = Bundle By Name(cluster=w355, "Anapana Start Time"=w353) -> (w354:T4)
        n142 = call <vilib>:"Add State(s) to Queue__JKI_lib_State_Machine.vi"("State(s) in (\"\")"=w358) -> ("States Out"=w357:string)  [unwired: 14 in]
      }
      frame "Timer: Check" {
        w373 = 60.0 ("y")
        # "Your code here.\n(You can make a copy of, or modify, this frame)"
        n143 = Unbundle By Name(w378) -> ("Anapana Start Time"=w376:timestamp, "Anapana"=w370:bool, "Vipassana"=w364:bool, "Anapana Time (min)"=w375:dbl, "Vipassana Time (min)"=w374:dbl)
        n144 = Get Date/Time In Seconds() -> (seconds since 1Jan1904=w377:timestamp)
        n145 = Subtract(x=w377, y=w376) -> (x-y=w366:dbl)
        n146 = Multiply(x=w375, y=w373) -> (x*y=w372:dbl)
        n147 = Multiply(x=w374, y=w373) -> (x*y=w365:dbl)
        n148 = Greater?(x=w366, y=w372) -> (0:w371:bool)
        n149 = Greater?(x=w366, y=w365) -> (0:w367:bool)
        n150 = And(x=w371, y=w370) -> (x .and. y?=w369:bool)
        n151 = And(x=w367, y=w364) -> (x .and. y?=w363:bool)
        n152 = Select(t="Bell Gongs: Single", s=w369, f="Timer: Wait\nTimer: Check") -> (s? t:f=w361:string)
        n153 = Select(t="Bell Gongs: Tripple", s=w363, f=w361) -> (s? t:f=w360:string)
        n154 = call <vilib>:"Add State(s) to Queue__JKI_lib_State_Machine.vi"("State(s) in (\"\")"=w381, "State(s) at Back (\"\")"=w360) -> ("States Out"=w380:string)  [unwired: 13 in]
      }
      frame "Timer: Stop" {
        # "Your code here.\n(You can make a copy of, or modify, this frame)"
        n155 = call <vilib>:"Add State(s) to Queue__JKI_lib_State_Machine.vi"("State(s) in (\"\")"=w385) -> ("States Out"=w384:string)  [unwired: 14 in]
      }
      frame "Timer: Wait" {
        # "Your code here.\n(You can make a copy of, or modify, this frame)"
        n156 = Wait (ms)(milliseconds to wait=u32 100) -> ()  [unwired: 1 out]
        n157 = call <vilib>:"Add State(s) to Queue__JKI_lib_State_Machine.vi"("State(s) in (\"\")"=w390) -> ("States Out"=w389:string)  [unwired: 14 in]
      }
    }
  }
